vi "CRYCalc Eq Wave for TSR.vi"(8 "EQ Rate":dbl format="%.2f", 9 "EQ Curve":T1={"Name"="", "Curve"=[], "X data"=1, "Y data"=1, "Z data"=1, "X axis"=0, "Y axis"=1, "Z axis"=1, "X unit"="Hz", "Y unit"="", "Z unit"="deg.", "X dB ref"=1.0, "Y dB ref"=1.0, "Z dB ref"=1.0, "single val"=FALSE, "protected"=FALSE, "display X"=TRUE, "display Y"=TRUE, "display Z"=TRUE, "Test Info"="", "Step No."=0, "Plot Settings"={"Color"=0, "Interpolation"=0, "Point Style"=0, "Line Style"=0, "Point Color"=0, "Line Width"=0, "Bar Plot Style"=0, "Fill To"=0}, "AutoProtect"=FALSE} {"Z data" items=["dB", "Lin"]; "X data" items=["dB", "Lin"]; "Y data" items=["dB", "Lin"]; "Z dB ref" format="%.1f"; "Z axis" items=["Log", "Lin"]; "X dB ref" format="%.1f"; "X axis" items=["Log", "Lin"]; "Y axis" items=["Log", "Lin"]; "Y dB ref" format="%.1f"; "Curve"."z" format="%.2f"; "Curve"."y" format="%.2f"; "Curve"."x" format="%.2f"}, 10 "Fs":dbl, 11 "Wave In":dbl[](array[numeric])) -> (2 "df":dbl, 3 "Wave Out":dbl[](array[numeric]))   [LabVIEW 2013]
uses:
  Typedef Control/CRYData Cluster.ctl
  <vilib>/Analysis/2dsp.llb/Real FFT.vi
  <vilib>/Analysis/2dsp.llb/Inverse Real FFT.vi
  <vilib>/Analysis/NI_AALPro.lvlib
panel:
  out "Waveform Graph 2":dbl[](graph)
  out "EQ":cluster{"x":dbl, "Lin Out":dbl}[](graph)
  out "Waveform Graph":dbl[](graph)
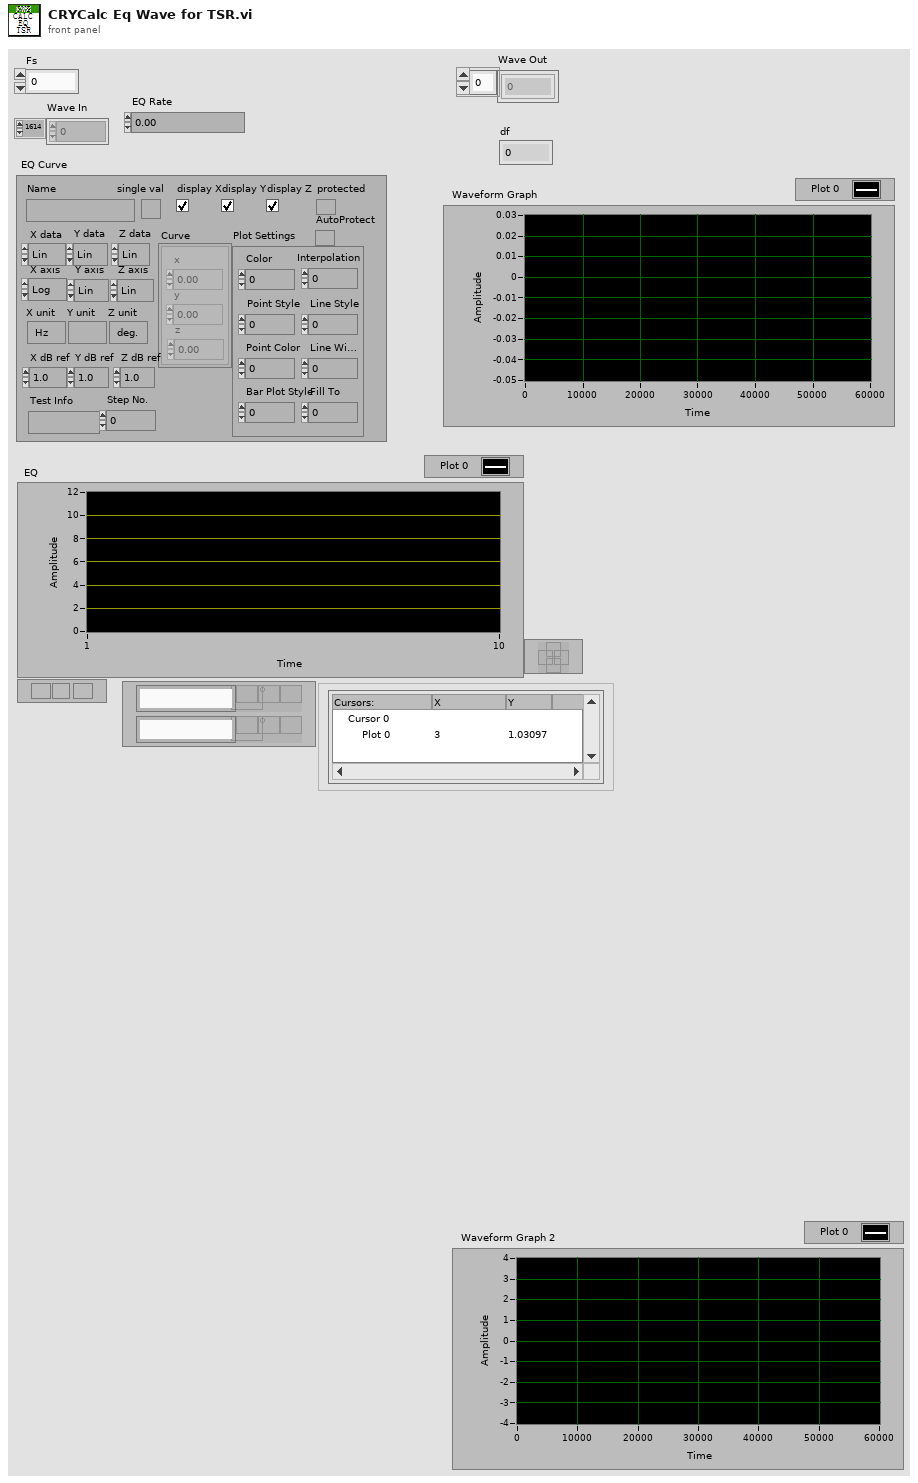
[diagram p1: front panel]
types:
  T1 = typedef "CRYData Cluster.ctl" = cluster{"Name":string, "Curve":cluster{"x":dbl, "y":dbl, "z":dbl}[], "X data":u16, "Y data":u16, "Z data":u16, "X axis":u16, "Y axis":u16, "Z axis":u16, "X unit":string, "Y unit":string, "Z unit":string, "X dB ref":dbl, "Y dB ref":dbl, "Z dB ref":dbl, "single val":bool, "protected":bool, "display X":bool, "display Y":bool, "display Z":bool, "Test Info":string, "Step No.":i32, "Plot Settings":cluster{"Color":u32, "Interpolation":u8, "Point Style":u8, "Line Style":u8, "Point Color":u32, "Line Width":u8, "Bar Plot Style":u8, "Fill To":i16}, "AutoProtect":bool}
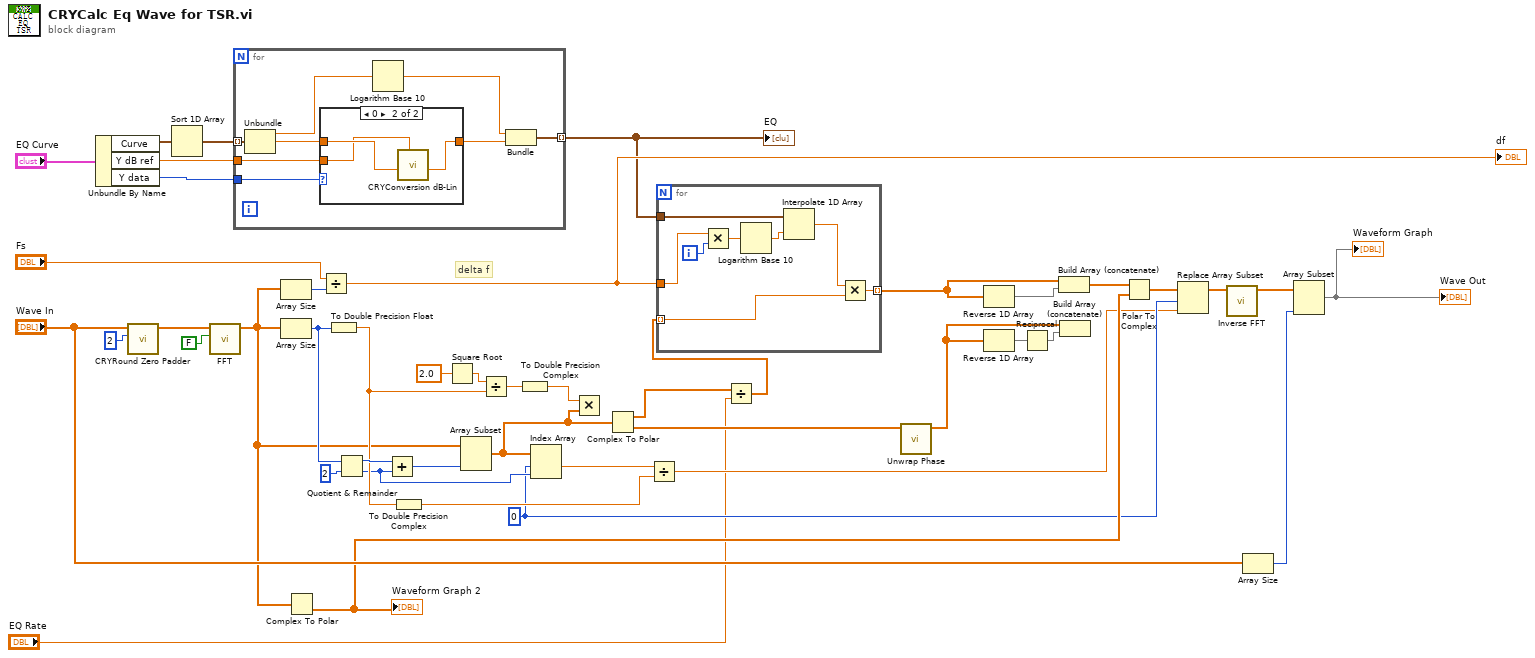
[diagram p0: block diagram]
diagram:
  w7 = 0 ("index")
  # "delta f"
  n1 = Unbundle By Name("EQ Curve") -> ("Curve"=w42:cluster{"x":dbl, "y":dbl, "z":dbl}[], "Y dB ref"=w41:dbl, "Y data"=w40:u16)
  n2 = call "CRYRound Zero Padder.vi"("Significant Digit"=u8 2, "Vector in"="Wave In") -> ("Zero Padder Vector out"=w22:dbl[])  [unwired: 8 in, 1 out]
  n3 = Sort 1D Array(array=w42) -> (sorted array=w10:cluster{"x":dbl, "y":dbl, "z":dbl}[])
  n4 = call-poly <vilib>:"FFT.vi"("shift?"=FALSE, "X"=w22) -> ("FFT {X}"=w17:cdb[])  [unwired: 8 in, 1 out]
  n5 = for {
    tunnel: w10 -> [w53] mode=indexing
    tunnel: [w52] -> w11 mode=indexing
    tunnel: w41 -> [w50]
    tunnel: w40 -> [w51]
    n6 = Unbundle(w53) -> ("x"=w47:dbl, "y"=w49:dbl)  [unwired: 1 out]
    n7 = case shown="0" w51 {
      tunnel: w49 -> [w54 w57]
      tunnel: [w54 w56] -> w48
      tunnel: w50 -> [_ w55]
      frame 1, Default {
      }
      frame 0 {
        n8 = call "CRYConversion dB-Lin.vi"("dB ref."=w55, "Log In"=w57) -> ("Lin Out"=w56:dbl)  [unwired: 4 in, 3 out]
      }
    }
    n9 = Logarithm Base 10(1:w47) -> (0:w46:dbl)
    n10 = Bundle(w46, "Lin Out"=w48) -> (w52:cluster{dbl, "Lin Out":dbl})  [unwired: 1 out]
  }
  "EQ" <- w11
  n11 = Array Size(array=w17) -> (size(s)=w39:i32)
  n12 = Array Size(array=w17) -> (size(s)=w32:i32)
  n13 = Complex To Polar(r * e^(i*theta)=w17) -> (theta=w14:dbl[])  [unwired: 1 out]
  "Waveform Graph 2" <- w14
  n14 = Divide(x="Fs", y=w39) -> (x/y=w29:dbl)
  "df" <- w29
  n15 = To Double Precision Float(number=w32) -> (double precision float=w31:dbl)
  n16 = Quotient & Remainder(x=w32, y=2) -> (x-y*floor(x/y)=w34:i32, floor(x/y)=w12:i32)
  n17 = Add(x=w34, y=w12) -> (x+y=w33:i32)
  n18 = To Double Precision Complex(1:w31) -> (0:w13:cdb)
  n19 = Square Root(x=2.0) -> (sqrt(x)=w24:dbl)
  n20 = Array Subset(array=w17, length=w33) -> (w18:cdb[])  [unwired: 1 in]
  n21 = Divide(x=w24, y=w31) -> (x/y=w23:dbl)
  n22 = To Double Precision Complex(1:w23) -> (0:w25:cdb)
  n23 = Index Array(array=w18, index #1=w7, index #2=w12) -> (element #1=w19:cdb)  [unwired: 1 out]
  n24 = Multiply(x=w25, y=w18) -> ()  [unwired: 1 out]
  n25 = Complex To Polar(r * e^(i*theta)=w18) -> (r=w3:dbl[], theta=w30:dbl[])
  n26 = Divide(x=w19, y=w13) -> (x/y=w6:cdb)
  n27 = Divide(x=w3, y="EQ Rate") -> (x/y=w2:dbl[])
  n28 = for {
    tunnel: w2 -> [w61] mode=indexing
    tunnel: w11 -> [w65]
    tunnel: [w64] -> w9 mode=indexing
    tunnel: w29 -> [w63]
    i -> [w62]
    n29 = Multiply(x=w63, y=w62) -> (x*y=w60:dbl)
    n30 = Logarithm Base 10(1:w60) -> (0:w59:dbl)
    n31 = Interpolate 1D Array(1:w59, 2:w65) -> (0:w58:dbl)
    n32 = Multiply(x=w58, y=w61) -> (x*y=w64:dbl)
  }
  n33 = call <vilib>:"Unwrap Phase.vi"("Phase"=w30) -> ("Unwrapped Phase"=w26:dbl[])  [unwired: 9 in, 1 out]
  n34 = Reverse 1D Array(array=w9) -> (reversed array=w28:dbl[])
  n35 = Reverse 1D Array(array=w26) -> (reversed array=w16:dbl[])
  n36 = Reciprocal(x=w16) -> (1/x=w15:dbl[])
  n37 = Build Array (concatenate)(w9, w28) -> (w27:dbl[])
  n38 = Build Array (concatenate)(w26, w15) -> ()  [unwired: 1 out]
  n39 = Polar To Complex(1:w14, 2:w27) -> (0:w8:cdb[])
  n40 = Replace Array Subset(array=w8, new element=w6, index=w7) -> (w5:cdb[])
  n41 = call-poly <vilib>:"Inverse FFT.vi"("FFT {X}"=w5) -> ("X"=w37:dbl[])  [unwired: 9 in, 1 out]
  n42 = Array Size(array="Wave In") -> (size(s)=w38:i32)
  n43 = Array Subset(array=w37, length=w38) -> (→"Wave Out" →"Waveform Graph":dbl[])  [unwired: 1 in]
